vi "Pulley.vi"() -> ()   [LabVIEW 2014]
uses:
  <vilib>/Rock Robotics/SystemInterfaces/Typedef/FPGA_TypedefDigitalModule.ctl
  <vilib>/Rock Robotics/SystemInterfaces/DIO/FPGA_DIOPWMChannel.ctl
  <vilib>/Rock Robotics/WPI/Joystick/WPI_JoystickDeviceEnum.ctl
  <vilib>/Rock Robotics/WPI/MotorControl/WPI_MotorControlOpen Talon.vi
panel:
  in  "stop":bool
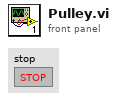
[diagram p1: front panel]
types:
  T1 = typedef "WPI_JoystickDeviceEnum.ctl" = enum16{"USB 0", "USB 1", "USB 2", "USB 3", "USB 4", "USB 5"}
  T2 = typedef "FPGA_DIOPWMChannel.ctl" = enum8{"PWM 0", "PWM 1", "PWM 2", "PWM 3", "PWM 4", "PWM 5", "PWM 6", "PWM 7", "PWM 8", "PWM 9", "PWM MXP 0", "PWM MXP 1", "PWM MXP 2", "PWM MXP 3", "PWM MXP 4", "PWM MXP 5", "PWM MXP 6", "PWM MXP 7", "PWM MXP 8", "PWM MXP 9", "Invalid"}
  T3 = typedef "FPGA_TypedefDigitalModule.ctl" = enum16{"Controller 1"}
  T4 = typedef "WPI_MotorControlDeviceRef.ctl" = cluster{"DeviceStatus":errorcluster, "Type":T5, "PWM":cluster{"Controller":T3, "PWM Channel":T2, "DeadBand":T6}, "CAN":cluster{"Device Number":u8, "Control Mode":T7, "Semaphore":T8, "Max Vout":dbl, "TalonSRX Control Mode":T9}, "Invert":bool, "TransformRef":T10, "InvTransformRef":T10}
  T5 = typedef "WPI_MotorControlType.ctl" = enum16{"PWM", "CAN", "CANTalonSRX"}
  T6 = typedef "WPI_PWMDeadband.ctl" = cluster{"Name":string, "maxPositivePwm":i32, "minPositivePwm":i32, "centerPwm":i32, "maxNegativePwm":i32, "minNegativePwm":i32, "angularRange":u16}
  T7 = typedef "WPI_CANJaguar_ControlMode.ctl" = enum8{"Percent VBus", "Current", "Speed", "Position", "Voltage"}
  T8 = typedef "Semaphore RefNum" = refnum<k1>
  T9 = typedef "WPI_CANTalonSRX_APIControlMode.ctl" = enum8{"Percent VBus", "Speed", "Position", "Slave", "Unchanged / Invalid"}
  T10 = typedef "WPI_PWMTransform_ConPane.ctl" = refnum<vi>
  T11 = typedef "WPI_JoystickDevRef.ctl" = cluster{"Device":T1}
  T12 = cluster{"Axes[0]":dbl, "Axes[1]":dbl, "Axes[2]":dbl, "Axes[3]":dbl, "Axes[4]":dbl, "Axes[5]":dbl, "Axes[6]":dbl, "Axes[7]":dbl, "Axes[8]":dbl}
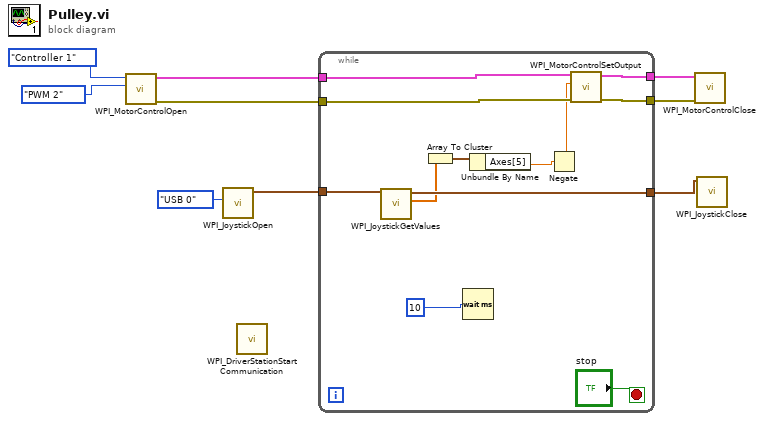
[diagram p0: block diagram]
diagram:
  n1 = call-poly <vilib>:"WPI_MotorControlOpen.vi"("PWM Channel"=FPGA_DIOPWMChannel."PWM 2", "Controller"=FPGA_TypedefDigitalModule."Controller 1") -> ("error out"=w2:errorcluster, "MotorControlDeviceRef"=w1:T4)  [unwired: 8 in]
  n2 = call <vilib>:"WPI_JoystickOpen.vi"("JoystickDevice"=WPI_JoystickDeviceEnum."USB 0") -> ("JoystickDevRef"=w6:T11)  [unwired: 10 in]
  n3 = call <vilib>:"WPI_DriverStationStart Communication.vi"() -> ()  [unwired: 12 in]
  n4 = while {
    tunnel: w6 -> [w21]
    tunnel: [w20] -> w3
    tunnel: [w18] -> w5
    tunnel: [w17] -> w4
    tunnel: w2 -> [w13]
    tunnel: w1 -> [w12]
    stop <- "stop" stop-if-true
    n5 = call <vilib>:"WPI_JoystickGetValues.vi"("JoystickDevRef"=w21) -> ("Axes"=w16:dbl[], "JoystickDevRef"=w20:T11)  [unwired: 6 in, 3 out]
    n6 = Array To Cluster(array=w16) -> (cluster=w15:T12)
    n7 = Wait (ms)(milliseconds to wait=10) -> ()  [unwired: 1 out]
    n8 = Unbundle By Name(w15) -> ("Axes[5]"=w11:dbl)
    n9 = Negate(x=w11) -> (-x=w10:dbl)
    n10 = call <vilib>:"WPI_MotorControlSetOutput.vi"("error in (no error)"=w13, "Output"=w10, "MotorControlDevRef"=w12) -> ("error out"=w17:errorcluster, "MotorControlDevRef"=w18:T4)  [unwired: 6 in, 1 out]
  }
  n11 = call <vilib>:"WPI_MotorControlClose.vi"("error in (no error)"=w4, "MotorControlDevRef"=w5) -> ()  [unwired: 9 in, 1 out]
  n12 = call <vilib>:"WPI_JoystickClose.vi"("JoystickDevRef"=w3) -> ()  [unwired: 11 in]
